vi "Can Elevator Test Code.vi"(11 "Joystick Input":dbl) -> ()   [LabVIEW 2014]
uses:
  <vilib>/Rock Robotics/WPI/CAN/TalonSRX/WPI_CANTalonSRX_GlobalStatus.ctl
panel:
  out "Added (Inverted) 2":bool
  out "Added (Inverted)":bool
  in  "Setpoint":dbl
  in  "PID Elevator 1":T1
  out "Talon SRX Status":T2
  in  "Setpoint 2":dbl
  in  "PID Elevator 2":T1
  out "Talon SRX Status 2":T2
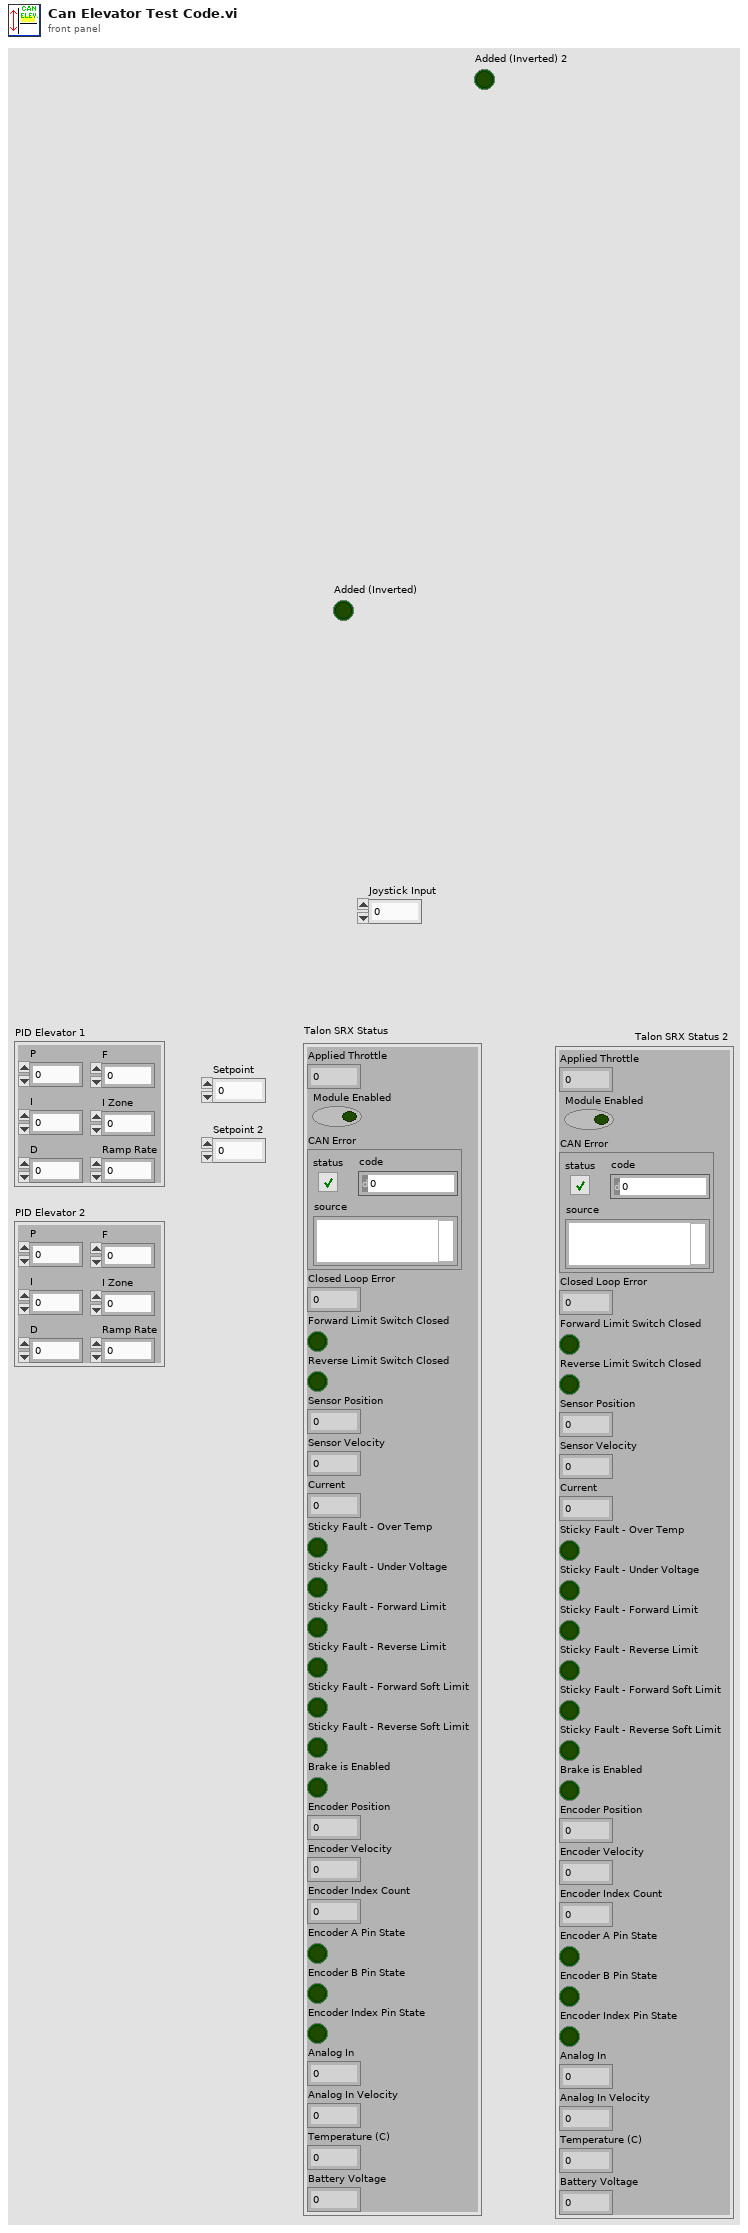
[diagram p1: front panel]
types:
  T1 = cluster{"P":dbl, "I":dbl, "D":dbl, "F":dbl, "I Zone":dbl, "Ramp Rate":dbl}
  T2 = typedef "WPI_CANTalonSRX_GlobalStatus.ctl" = cluster{"Applied Throttle":dbl, "Module Enabled":bool, "CAN Error":errorcluster, "Closed Loop Error":dbl, "Forward Limit Switch Closed":bool, "Reverse Limit Switch Closed":bool, "Sensor Position":dbl, "Sensor Velocity":dbl, "Current":dbl, "Sticky Fault - Over Temp":bool, "Sticky Fault - Under Voltage":bool, "Sticky Fault - Forward Limit":bool, "Sticky Fault - Reverse Limit":bool, "Sticky Fault - Forward Soft Limit":bool, "Sticky Fault - Reverse Soft Limit":bool, "Brake is Enabled":bool, "Encoder Position":dbl, "Encoder Velocity":dbl, "Encoder Index Count":dbl, "Encoder A Pin State":bool, "Encoder B Pin State":bool, "Encoder Index Pin State":bool, "Analog In":dbl, "Analog In Velocity":dbl, "Temperature (C)":dbl, "Battery Voltage":dbl}
  T3 = typedef "WPI_MotorControlDeviceRef.ctl" = cluster{"DeviceStatus":errorcluster, "Type":T4, "PWM":cluster{"Controller":T5, "PWM Channel":T6, "DeadBand":T7}, "CAN":cluster{"Device Number":u8, "Control Mode":T8, "Semaphore":T9, "Max Vout":dbl, "TalonSRX Control Mode":T10}, "Invert":bool, "TransformRef":T11, "InvTransformRef":T11}
  T4 = typedef "WPI_MotorControlType.ctl" = enum16{"PWM", "CAN", "CANTalonSRX"}
  T5 = typedef "FPGA_TypedefDigitalModule.ctl" = enum16{"Controller 1"}
  T6 = typedef "FPGA_DIOPWMChannel.ctl" = enum8{"PWM 0", "PWM 1", "PWM 2", "PWM 3", "PWM 4", "PWM 5", "PWM 6", "PWM 7", "PWM 8", "PWM 9", "PWM MXP 0", "PWM MXP 1", "PWM MXP 2", "PWM MXP 3", "PWM MXP 4", "PWM MXP 5", "PWM MXP 6", "PWM MXP 7", "PWM MXP 8", "PWM MXP 9", "Invalid"}
  T7 = typedef "WPI_PWMDeadband.ctl" = cluster{"Name":string, "maxPositivePwm":i32, "minPositivePwm":i32, "centerPwm":i32, "maxNegativePwm":i32, "minNegativePwm":i32, "angularRange":u16}
  T8 = typedef "WPI_CANJaguar_ControlMode.ctl" = enum8{"Percent VBus", "Current", "Speed", "Position", "Voltage"}
  T9 = typedef "Semaphore RefNum" = refnum<k1>
  T10 = typedef "WPI_CANTalonSRX_APIControlMode.ctl" = enum8{"Percent VBus", "Speed", "Position", "Slave", "Unchanged / Invalid"}
  T11 = typedef "WPI_PWMTransform_ConPane.ctl" = refnum<vi>
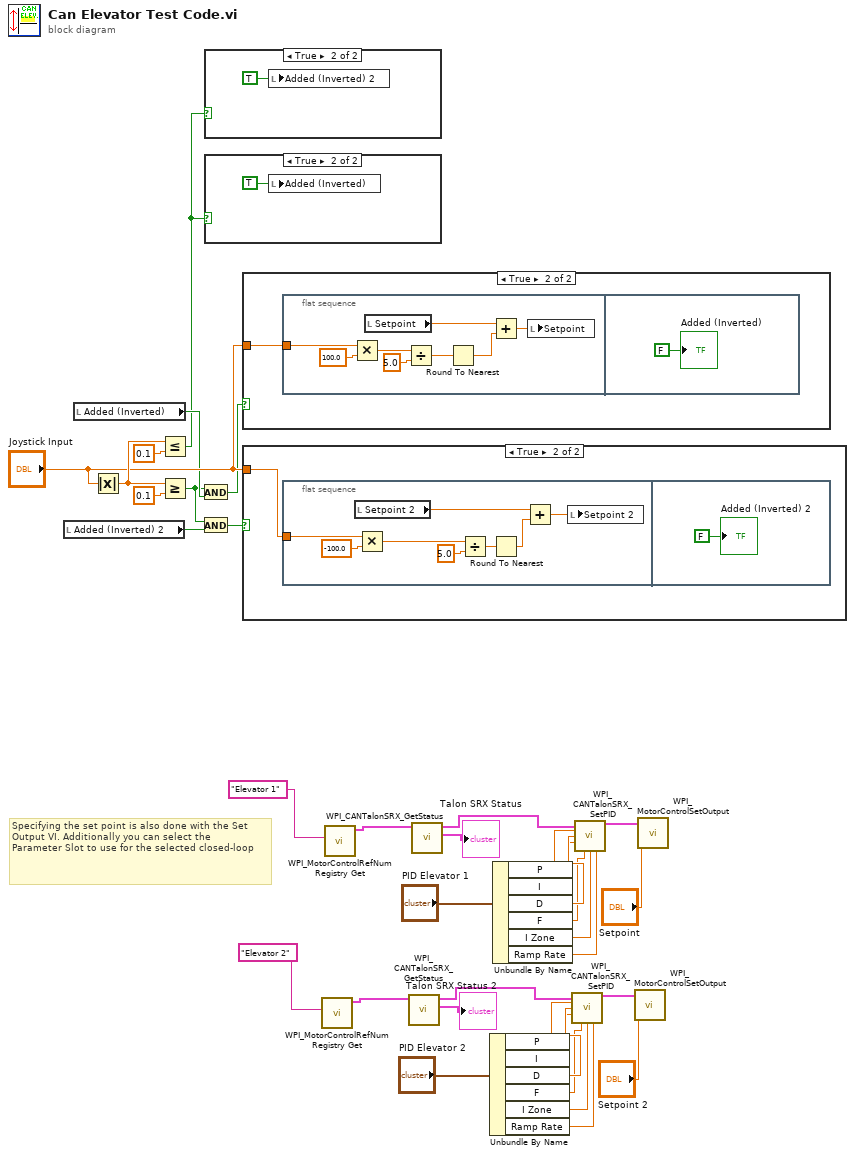
[diagram p0: block diagram]
diagram:
  # "Specifying the set point is also done with the Set Output VI. Additionally you can select the\nParameter Slot to use for the selected closed-loop"
  n1 = local read "Added (Inverted) 2"() -> (w4:bool)
  n2 = local read "Added (Inverted)"() -> (w5:bool)
  n3 = Absolute Value(x="Joystick Input") -> (abs(x)=w8:dbl)
  n4 = Less Or Equal?(x=w8, y=0.1) -> (x <= y?=w2:bool)
  n5 = Greater Or Equal?(x=w8, y=0.1) -> (x >= y?=w1:bool)
  n6 = And(x=w1, y=w5) -> (x .and. y?=w6:bool)
  n7 = And(x=w1, y=w4) -> (x .and. y?=w3:bool)
  n8 = case shown="True" w2 {
    frame False {
    }
    frame True {
      n9 = local write "Added (Inverted) 2"(TRUE) -> ()
    }
  }
  n10 = case shown="True" w2 {
    frame False {
    }
    frame True {
      n11 = local write "Added (Inverted)"(TRUE) -> ()
    }
  }
  n12 = case shown="True" w6 {
    tunnel: "Joystick Input" -> [_ w39]
    frame False {
    }
    frame True {
      n13 = flat-sequence {
        tunnel: w39 -> [w43]
        frame #0 {
          n14 = Multiply(x=w43, y=100.0) -> (x*y=w46:dbl)
          n15 = local read "Setpoint"() -> (w41:dbl)
          n16 = Divide(x=w46, y=5.0) -> (x/y=w44:dbl)
          n17 = Round To Nearest(number=w44) -> (nearest integer value=w42:dbl)
          n18 = Add(x=w41, y=w42) -> (x+y=w40:dbl)
          n19 = local write "Setpoint"(w40) -> ()
        }
        frame #1 {
          "Added (Inverted)" <- FALSE
        }
      }
    }
  }
  n20 = case shown="True" w3 {
    tunnel: "Joystick Input" -> [_ w49]
    frame False {
    }
    frame True {
      n21 = flat-sequence {
        tunnel: w49 -> [w53]
        frame #0 {
          n22 = local read "Setpoint 2"() -> (w51:dbl)
          n23 = Multiply(x=w53, y=-100.0) -> (x*y=w56:dbl)
          n24 = Divide(x=w56, y=5.0) -> (x/y=w54:dbl)
          n25 = Round To Nearest(number=w54) -> (nearest integer value=w52:dbl)
          n26 = Add(x=w51, y=w52) -> (x+y=w50:dbl)
          n27 = local write "Setpoint 2"(w50) -> ()
        }
        frame #1 {
          "Added (Inverted) 2" <- FALSE
        }
      }
    }
  }
  n28 = call <vilib>:"WPI_MotorControlRefNum Registry Get.vi"("refnum name"="Elevator 2") -> ("MotorControlDevRef"=w36:T3)  [unwired: 9 in, 1 out]
  n29 = call <vilib>:"WPI_MotorControlRefNum Registry Get.vi"("refnum name"="Elevator 1") -> ("MotorControlDevRef"=w23:T3)  [unwired: 9 in, 1 out]
  n30 = call <vilib>:"WPI_CANTalonSRX_GetStatus.vi"("CAN Talon SRX Ref"=w36) -> ("Talon SRX Status"=→"Talon SRX Status 2":T2, "CAN Talon SRX Ref Out"=w33:T3)  [unwired: 8 in, 1 out]
  n31 = call <vilib>:"WPI_CANTalonSRX_GetStatus.vi"("CAN Talon SRX Ref"=w23) -> ("Talon SRX Status"=→"Talon SRX Status":T2, "CAN Talon SRX Ref Out"=w20:T3)  [unwired: 8 in, 1 out]
  n32 = Unbundle By Name("PID Elevator 2") -> ("P"=w31:dbl, "I"=w30:dbl, "D"=w29:dbl, "F"=w28:dbl, "I Zone"=w27:dbl, "Ramp Rate"=w26:dbl)
  n33 = Unbundle By Name("PID Elevator 1") -> ("P"=w18:dbl, "I"=w17:dbl, "D"=w16:dbl, "F"=w15:dbl, "I Zone"=w14:dbl, "Ramp Rate"=w13:dbl)
  n34 = call <vilib>:"WPI_CANTalonSRX_SetPID.vi"("CAN Talon SRX Ref"=w33, "P"=w31, "I"=w30, "D"=w29, "F"=w28, "I Zone"=w27, "Ramp Rate"=w26) -> ("CAN Talon SRX Ref Out"=w24:T3)  [unwired: 7 in, 1 out]
  n35 = call <vilib>:"WPI_CANTalonSRX_SetPID.vi"("CAN Talon SRX Ref"=w20, "P"=w18, "I"=w17, "D"=w16, "F"=w15, "I Zone"=w14, "Ramp Rate"=w13) -> ("CAN Talon SRX Ref Out"=w11:T3)  [unwired: 7 in, 1 out]
  n36 = call <vilib>:"WPI_MotorControlSetOutput.vi"("Output"="Setpoint 2", "MotorControlDevRef"=w24) -> ()  [unwired: 7 in, 3 out]
  n37 = call <vilib>:"WPI_MotorControlSetOutput.vi"("Output"="Setpoint", "MotorControlDevRef"=w11) -> ()  [unwired: 7 in, 3 out]
